vi "Read Factory Parameters.vi"(0 "Session Handle in":T1, 5 "Address":u8, 11 "error in (no error)":errorcluster) -> (4 "Session Handle out":T1, 6 "Read Bytes":u8[](array[numeric]), 15 "error out":errorcluster)   [LabVIEW 2015, in "Oil.lvclass"]
uses:
  Oil.lvclass
  Typedefs/Session Handle.ctl
panel:
  out "Whole Payload":u8[](array[numeric])
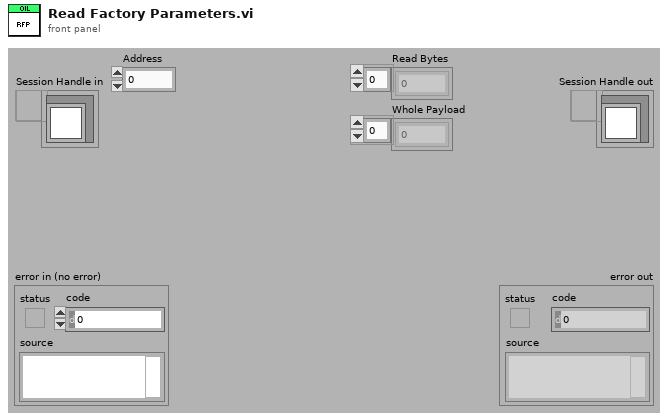
[diagram p1: front panel]
types:
  T1 = typedef "Oil.lvclass/Session Handle.ctl" = refnum<data-value>
  T2 = typedef "XNET Frame CAN.ctl" = cluster{"timestamp":timestamp, "payload":u8[], "identifier":u32, "type":T3, "extended?":bool, "echo?":bool}
  T3 = typedef "XNET Frame Type CAN.ctl" = u8
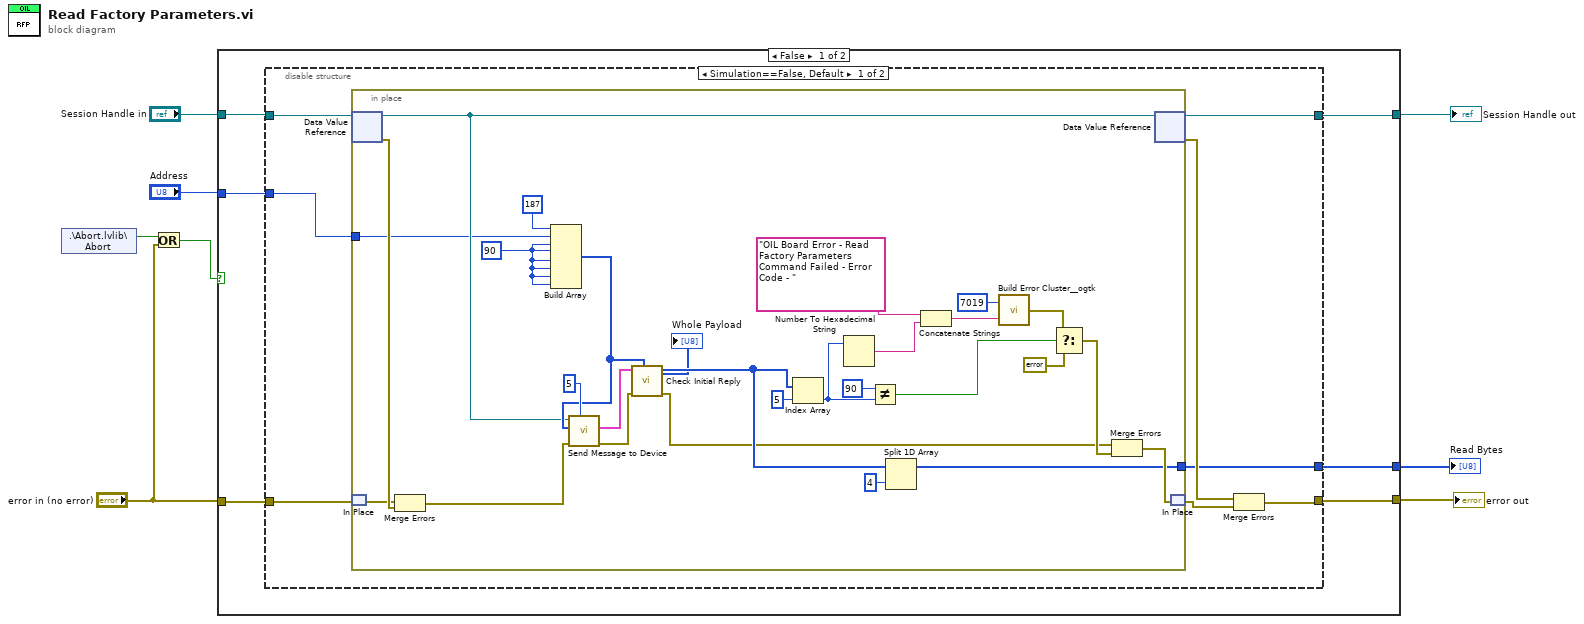
[diagram p0: block diagram]
diagram:
  n1 = shared-variable ".\\Abort.lvlib\\Abort"() -> (w5:bool)  [unwired: 1 in, 1 out]
  n2 = Or(x=w5, y="error in (no error)") -> (x .or. y?=w4:bool)
  n3 = case shown="False" w4 {
    tunnel: "Session Handle in" -> [w14 w54]
    tunnel: [w13 w54] -> w7
    tunnel: [w12 w53] -> w6
    tunnel: "error in (no error)" -> [w11 w53]
    tunnel: "Address" -> [w10 _]
    tunnel: [w9 _] -> w1
    frame False {
      n4 = disable-structure shown="Simulation==False, Default" {
        disable-tunnel: w14 -> [w22 w52]
        disable-tunnel: [w21 w52] -> w13
        disable-tunnel: [w19 w51] -> w12
        disable-tunnel: w11 -> [w20 w51]
        disable-tunnel: w10 -> [w16 _]
        disable-tunnel: [w15 _] -> w9
        frame condition #0 (active) {
          n5 = in-place {
            in-place-border: w16 -> [w25]
            in-place-border: [w24] -> w15
            w34 = u8 90
            n6 = in-place-dvr #1(w22) -> (w29:refnum<class "Oil.lvclass">, w50:errorcluster)
            n7 = in-place-match #2(w20) -> (w49:errorcluster)
            n8 = Merge Errors(w49, w50) -> (w28:errorcluster)
            n9 = Build Array(u8 187, w25, w34, w34, w34, w34, w34, w34) -> (w31:u8[])
            n10 = call "Send Message to Device.vi"("Number of Retries"=5, "error in (no error)"=w28, "payload"=w31, "CAN Comm In"=w29) -> ("error out"=w32:errorcluster, "Reply"=w33:T2[])  [unwired: 5 in, 1 out]
            n11 = call "Check Initial Reply.vi"("Write Message"=w31, "error in (no error)"=w32, "Reply"=w33) -> ("error out"=w27:errorcluster, "Data Packet 2"=w30:u8[], "Whole Payload"=→"Whole Payload":u8[])  [unwired: 5 in, 1 out]
            n12 = Index Array(array=w30, index=5) -> (element=w40:u8)
            n13 = Number To Hexadecimal String(2:w40) -> (0:w39:string)  [unwired: 1 in]
            n14 = Not Equal?(x=u8 90, y=w40) -> (x != y?=w37:bool)
            n15 = Split 1D Array(array=w30, index=4) -> (first subarray=w24:u8[])  [unwired: 1 out]
            n16 = Concatenate Strings("OIL Board Error - Read Factory Parameters Command Failed - Error Code - " ("string"), w39) -> (w38:string)
            n17 = call <userlib>:"Build Error Cluster__ogtk.vi"("String to Prepend to source (\"\")"=w38, "code"=7019) -> ("error out"=w46:errorcluster)
            n18 = Select(t=w46, s=w37, f=errorcluster {"status"=FALSE, "code"=0, "source"=""}) -> (s? t:f=w36:errorcluster)
            n19 = Merge Errors(w27, w36) -> (w26:errorcluster)
            n20 = in-place-dvr #1(w29) -> (w21:T1, w17:errorcluster)
            n21 = in-place-match #2(w26) -> (w18:errorcluster)
          }
          n22 = Merge Errors(w17, w18) -> (w19:errorcluster)
        }
        frame condition #1 {
        }
      }
    }
    frame True {
    }
  }
  "Session Handle out" <- w7
  "error out" <- w6
  "Read Bytes" <- w1
